vi "XY Graph Replace Single Plot.vi"(0 "XYGraph Ref in":T3, 2 "Plot Interpolation (Previous Plot's Style)":T2=enum."Use Previous Plot's Style", 5 "Plot":cluster{"X Array":dbl[], "Y Array":dbl[]}, 7 "Plot index":i32, 9 "Plot Name (\"Plot\")":string, 11 "error in (no error)":errorcluster, 12 "Plot Metadata":variant, 13 "Plot Color (Default)":u32(colorbox)=15781887, 14 "Point Style (Dot)":T1=enum."Dot") -> (4 "XY Graph Caption (or Label)":string, 8 "Plot Index":i32, 10 "Plot Name":string, 15 "error out":errorcluster)   [LabVIEW 2021, in "XY Graph Add-Ons.lvlib"]
uses:
  XY Graph Add-Ons.lvlib
  XY Graph Refnum.ctl
  LabVIEW Plot Interpolation.ctl
  Plot Point Style.ctl
  Plot Magic Color (Unchanged).ctl
  XY Graph Get Plots Metadata.vi
  XY Graph Set Plots Metadata.vi
  Strings/Strings.lvlib
  Graphs.lvlib
  Error/Error.lvlib
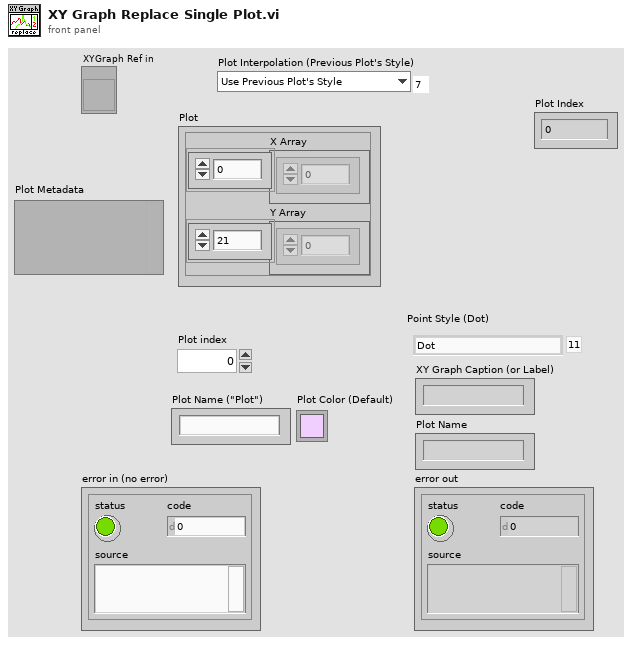
[diagram p1: front panel]
types:
  T1 = typedef "Graphs.lvlib/Plot Point Style.ctl" = enum16{"not defined", "None", "Empty Circle", "Filled Circle", "Thick Circle", "Dotted Circle", "Empty Square", "Filled Square", "Thick Square", "Dotted Square", "Small Filled Square", "Dot", "Cross", "Tiny Cross", "Large X", "Small x", "Diamond", "Small Empty Square"}
  T2 = typedef "Graphs.lvlib/LabVIEW Plot Interpolation.ctl" = enum16{"Point (.)", "Stepwise Right (--.)", "Line + Point (\\. /)", "Stepwise Left (.--)", "Stepwise Centered (-.-)", "Stepwise Vertical (|.|)", "Line (-)", "Use Previous Plot's Style"}
  T3 = typedef "XY Graph Add-Ons.lvlib/XY Graph Refnum.ctl" = refnum<vi>
  T4 = typedef "Graphs.lvlib/Plot Magic Color (Unchanged).ctl" = u32
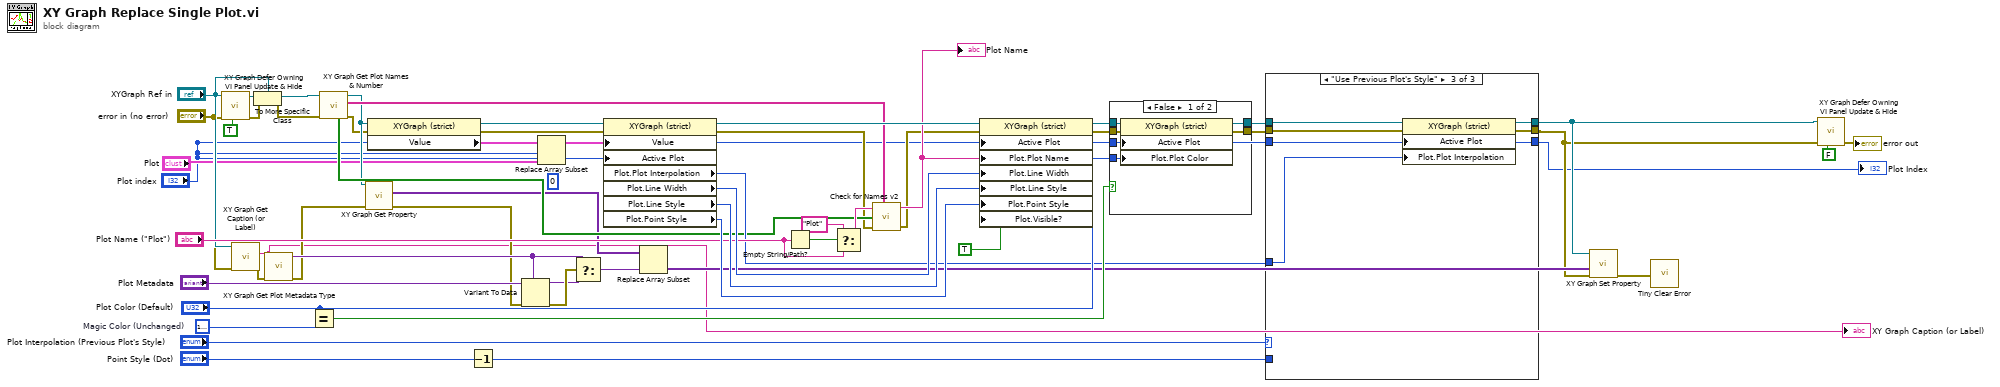
[diagram p0: block diagram]
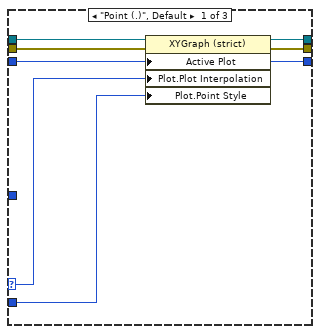
[diagram p2: hidden frame]
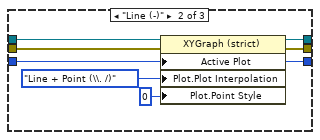
[diagram p3: hidden frame]
diagram:
  (unwired) 0 ("y")
  w47 = T4 15781887  # Magic Color (Unchanged)
  n1 = call "XY Graph Defer Owning VI Panel Update & Hide.vi"("Defer Owning Panel Update"=TRUE, "error in (no error)"="error in (no error)", "XY Graph Refnum in"="XYGraph Ref in") -> ("error out"=w24:errorcluster, "XY Graph Refnum out"=w30:refnum<vi>)  [unwired: 7 in]
  n2 = call "XY Graph Get Caption (or Label).vi"("error in (no error)"="error in (no error)", "XY Graph in"="XYGraph Ref in") -> ("error out"=w10:errorcluster, "Caption (or Label) Text"=w9:string)  [unwired: 7 in, 1 out]
  "XY Graph Caption (or Label)" <- w9
  n3 = To More Specific Class(target class="XYGraph Ref in", reference=w30, error in=w24) -> (specific class reference=w25:T3, error out=w23:errorcluster)
  n4 = call "XY Graph Get Plot Metadata Type.vi"("Error In"=w10, "Graph Label"=w9) -> ("Error Out"=w13:errorcluster, "Plot Metadata Type"=w15:variant)  [unwired: 7 in, 1 out]
  n5 = Equal?(x="Plot Color (Default)", y=w47) -> (x = y?=w44:bool)
  n6 = call "XY Graph Get Plot Names & Number.vi"("error in (no error)"=w23, "XYGraph in"=w25) -> ("error out"=w6:errorcluster, "Plot Names"=w35:string[], "XYGraph out"=w7:T3, "Empty Plots?"=w28:bool[])  [unwired: 4 in, 2 out]
  n7 = call-poly "XY Graph Get Property.vi"("Error In"=w13, "XYGraph Ref"=w7) -> ("Error Out"=w12:errorcluster, "Plot Metadata"=w21:variant[])  [unwired: 6 in, 2 out]
  n8 = property class="XYGraph (strict)"(reference=w7, error in=w6) -> (reference out=w56:T3, error out=w38:errorcluster, "Value"=w54:cluster{"X Array":dbl[], "Y Array":dbl[]}[])
  n9 = Decrement(x="Point Style (Dot)") -> (x-1=w32:T1)
  n10 = Variant To Data(error in=w12, type=w15, Variant="Plot Metadata") -> (data=w14:variant, error out=w16:errorcluster)
  n11 = Replace Array Subset(array=w54, new element="Plot", index="Plot index") -> (w57:cluster{"X Array":dbl[], "Y Array":dbl[]}[])
  n12 = Select(t=w15, s=w16, f=w14) -> (s? t:f=w8:variant)
  n13 = property class="XYGraph (strict)"(reference=w56, error in=w38, "Value"=w57, "Active Plot"="Plot index") -> (reference out=w55:T3, error out=w27:errorcluster, "Plot.Plot Interpolation"=w39:u8, "Plot.Line Width"=w53:u8, "Plot.Line Style"=w52:u8, "Plot.Point Style"=w51:u8)
  n14 = Replace Array Subset(array=w21, new element=w8) -> (w20:variant[])  [unwired: 1 in]
  n15 = Empty String/Path?(string/path="Plot Name (\"Plot\")") -> (empty?=w50:bool)
  n16 = Select(t="Plot", s=w50, f="Plot Name (\"Plot\")") -> (s? t:f=w34:string)
  n17 = call "Check for Names v2.vi"("New Name"=w34, "Name List"=w35, "Empty Plots?"=w28, "Error In"=w27) -> ("New Name"=w33:string, "Error Out"=w26:errorcluster)  [unwired: 2 in, 2 out]
  "Plot Name" <- w33
  n18 = property class="XYGraph (strict)"(reference=w55, error in=w26, "Active Plot"="Plot index", "Plot.Plot Name"=w33, "Plot.Line Width"=w53, "Plot.Line Style"=w52, "Plot.Point Style"=w51, "Plot.Visible?"=TRUE ("Plot.Visible")) -> (reference out=w46:T3, error out=w45:errorcluster)
  n19 = case shown="False" w44 {
    tunnel: w46 -> [w63 w65]
    tunnel: [w62 w65] -> w42
    tunnel: w45 -> [w61 w64]
    tunnel: [w60 w64] -> w41
    tunnel: "Plot index" -> [w59 _]
    tunnel: "Plot Color (Default)" -> [w58 _]
    frame False {
      n20 = property class="XYGraph (strict)"(reference=w63, error in=w61, "Active Plot"=w59, "Plot.Plot Color"=w58) -> (reference out=w62:T3, error out=w60:errorcluster)
    }
    frame True {
    }
  }
  n21 = case shown="\"Use Previous Plot's Style\"" "Plot Interpolation (Previous Plot's Style)" {
    selector: "Plot Interpolation (Previous Plot's Style)" -> [w68 _ _]
    tunnel: w42 -> [w72 w79 w85]
    tunnel: [w71 w78 w84] -> w3
    tunnel: w41 -> [w70 w77 w83]
    tunnel: [w69 w76 w82] -> w2
    tunnel: "Plot index" -> [w66 w73 w80]
    tunnel: w39 -> [_ _ w81]
    tunnel: w32 -> [w67 _ _]
    tunnel: [w66 w73 w80] -> w1
    frame "Point (.)", Default {
      n22 = property class="XYGraph (strict)"(reference=w72, error in=w70, "Active Plot"=w66, "Plot.Plot Interpolation"=w68, "Plot.Point Style"=w67) -> (reference out=w71:T3, error out=w69:errorcluster)
    }
    frame "Line (-)" {
      n23 = property class="XYGraph (strict)"(reference=w79, error in=w77, "Active Plot"=w73, "Plot.Plot Interpolation"=LabVIEW_Plot_Interpolation."Line + Point (\\. /)" ("Plot Interpolation (Previous Plot's Style)"), "Plot.Point Style"=u8 0) -> (reference out=w78:T3, error out=w76:errorcluster)
    }
    frame "Use Previous Plot's Style" {
      n24 = property class="XYGraph (strict)"(reference=w85, error in=w83, "Active Plot"=w80, "Plot.Plot Interpolation"=w81) -> (reference out=w84:T3, error out=w82:errorcluster)
    }
  }
  "Plot Index" <- w1
  n25 = call-poly "XY Graph Set Property.vi"("error in (no error)"=w2, "Plots Metadata"=w20, "XY Graph Refnum"=w3) -> ("error out"=w19:errorcluster)  [unwired: 7 in, 1 out]
  n26 = call "Tiny Clear Error.vi"("Error In"=w19) -> ()  [unwired: 8 in, 1 out]
  n27 = call "XY Graph Defer Owning VI Panel Update & Hide.vi"("Defer Owning Panel Update"=FALSE, "error in (no error)"=w2, "XY Graph Refnum in"=w3) -> ("error out"=→"error out":errorcluster)  [unwired: 7 in, 1 out]
